vi "Ball Trajectory.vi"(11 "Distance Away (x)":dbl) -> (2 "Angle":dbl, 3 "Speed of ball leaving flywheel":dbl)   [LabVIEW 2019]
panel:
  out "XY Graph":cluster{"X":dbl, "Y":dbl}[](graph)
  # "Requirements: Passes through goal at exactly the top of the arc"
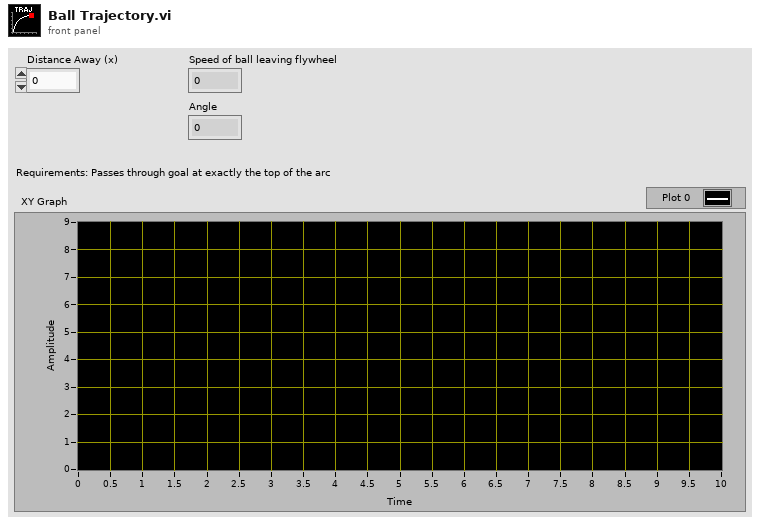
[diagram p1: front panel]
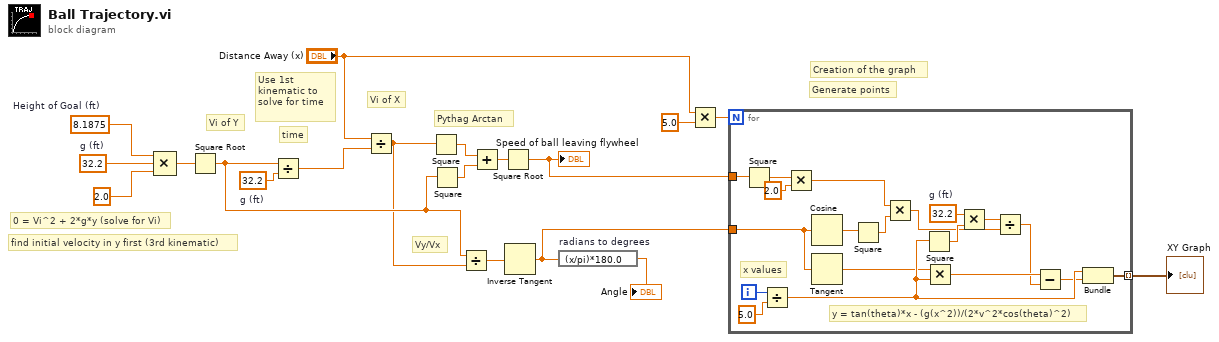
[diagram p0: block diagram]
diagram:
  w15 = 32.2  # g (ft)
  w18 = 32.2  # g (ft)
  w19 = 8.1875  # Height of Goal (ft)
  # "Generate points"
  # "Creation of the graph"
  # "Vy/Vx"
  # "Pythag Arctan"
  # "Vi of X"
  # "time"
  # "Use 1st kinematic to solve for time"
  # "Vi of Y"
  # "0 = Vi^2 + 2*g*y (solve for Vi)"
  # "find initial velocity in y first (3rd kinematic)"
  n1 = Compound Arithmetic op=MULTIPLY(w19, w18, 2.0 ("value")) -> (w16:dbl)
  n2 = Square Root(x=w16) -> (sqrt(x)=w9:dbl)
  n3 = Divide(x=w9, y=w15) -> (x/y=w10:dbl)
  n4 = Divide(x="Distance Away (x)", y=w10) -> (x/y=w1:dbl)
  n5 = Square(x=w1) -> (x^2=w13:dbl)
  n6 = Square(x=w9) -> (x^2=w14:dbl)
  n7 = Divide(x=w9, y=w1) -> (x/y=w11:dbl)
  n8 = Add(x=w13, y=w14) -> (x+y=w12:dbl)
  n9 = Square Root(x=w12) -> (sqrt(x)=w3:dbl)
  "Speed of ball leaving flywheel" <- w3
  n10 = Inverse Tangent(1:w11) -> (0:w4:dbl)
  n11 = expression code="(x/pi)*180.0" "radians to degrees"(w4) -> (→"Angle":dbl)
  n12 = Multiply(x="Distance Away (x)", y=5.0) -> (x*y=w8:dbl)
  n13 = for {
    N: w8 -> [_]
    tunnel: w4 -> [w30]
    tunnel: w3 -> [w32]
    tunnel: [w22] -> w2 mode=indexing
    i -> [w38]
    w36 = 32.2  # g (ft)
    # "y = tan(theta)*x - (g(x^2))/(2*v^2*cos(theta)^2)"
    # "x values"
    n14 = Square(x=w32) -> (x^2=w31:dbl)
    n15 = Divide(x=w38, y=5.0) -> (x/y=w24:dbl)
    n16 = Multiply(x=w31, y=2.0) -> (x*y=w28:dbl)
    n17 = Cosine(x=w30) -> (cos(x)=w21:dbl)
    n18 = Tangent(1:w30) -> (0:w20:dbl)
    n19 = Square(x=w21) -> (x^2=w29:dbl)
    n20 = Multiply(x=w28, y=w29) -> (x*y=w27:dbl)
    n21 = Square(x=w24) -> (x^2=w35:dbl)
    n22 = Multiply(x=w20, y=w24) -> (x*y=w26:dbl)
    n23 = Multiply(x=w36, y=w35) -> (x*y=w34:dbl)
    n24 = Divide(x=w34, y=w27) -> (x/y=w25:dbl)
    n25 = Subtract(x=w26, y=w25) -> (x-y=w23:dbl)
    n26 = Bundle(w24, w23) -> (w22:cluster{dbl, dbl})  [unwired: 1 in]
  }
  "XY Graph" <- w2
